vi "ep_Build Waveforms.vi"(0 "AI data":sgl[][](array[numeric]) format="%#.21g", 1 "wiring":T1, 2 "reset? (F)":bool, 5 "AI data channel order":T2[](array[typedef])=[enum."Voltage Phase A (L1)", enum."Voltage Phase B (L2)", enum."Voltage Phase C (L3)", enum."Current Phase A (L1)", enum."Current Phase B (L2)", enum."Current Phase C (L3)", enum."Current Phase N (Neutral)"], 7 "dt":dbl, 9 "t0":timestamp, 11 "error in (no error)":errorcluster) -> (4 "voltage waveforms":waveform(sgl)[](array[waveform]), 6 "current waveforms":waveform(sgl)[](array[waveform]), 15 "error out":errorcluster)   [LabVIEW 2011, in "NI_EP_Power Quality.lvlib"]
uses:
  <vilib>/addons/Electrical Power/PQ/NI_EP_Power Quality.lvlib
  <vilib>/addons/Electrical Power/PQ/Common/Controls/ep_AI Data Channel.ctl
  <vilib>/addons/Electrical Power/PQ/Common/Controls/ep_Wiring.ctl
  <vilib>/addons/Electrical Power/PQ/Scaling_Calibration/subVIs/ep_Compute Third Current (SGL WFM).vi
panel:
  in  "waveform":waveform(sgl)
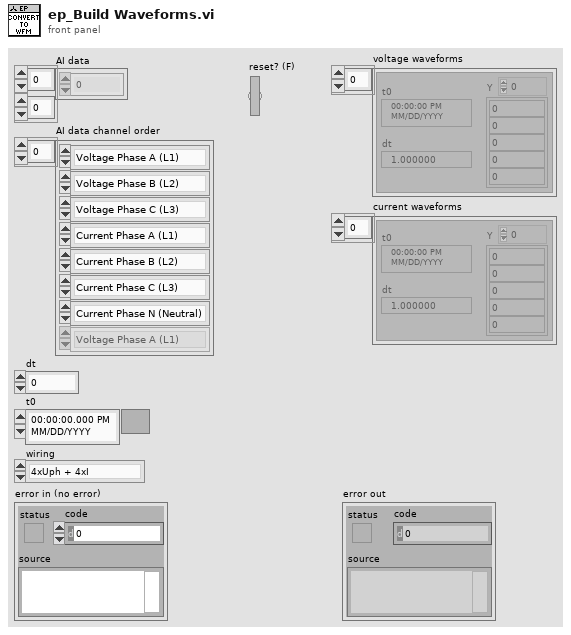
[diagram p1: front panel]
types:
  T1 = typedef "NI_EP_Power Quality.lvlib/ep_Wiring.ctl" = enum16{"4xUph + 4xI", "3xUph + 4xI", "3xUline + 4xI", "3xUph + 3xI", "3xUline + 3xI", "3xUph + 2xI", "3xUline + 2xI", "1xUph + 1xI"}
  T2 = typedef "NI_EP_Power Quality.lvlib/ep_AI Data Channel.ctl" = enum16{"Voltage Phase A (L1)", "Voltage Phase B (L2)", "Voltage Phase C (L3)", "Voltage Phase N (Neutral)", "Current Phase A (L1)", "Current Phase B (L2)", "Current Phase C (L3)", "Current Phase N (Neutral)"}
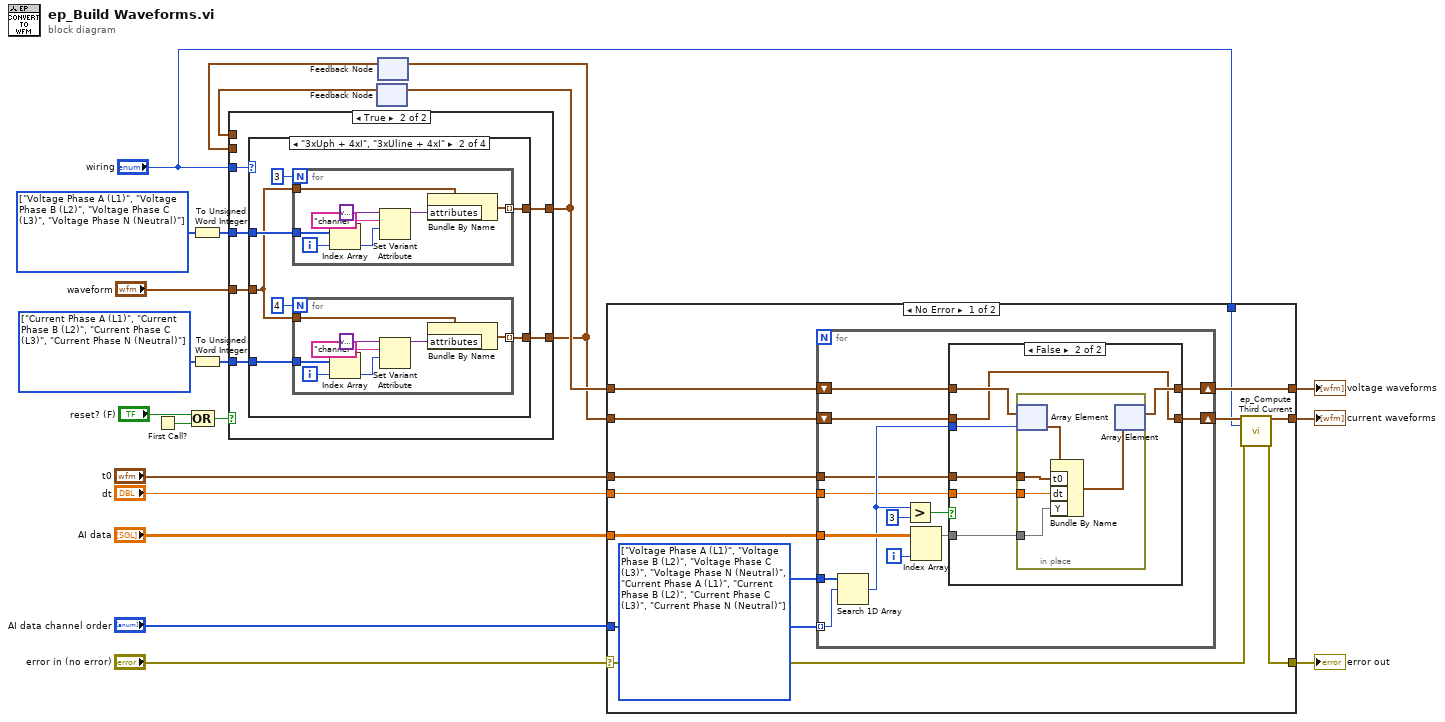
[diagram p0: block diagram]
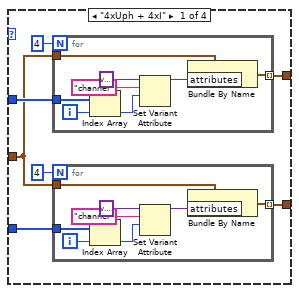
[diagram p3: hidden frame]
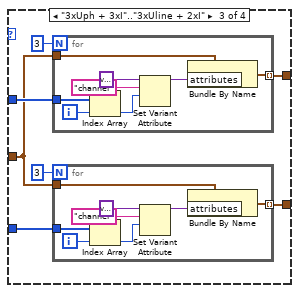
[diagram p4: hidden frame]
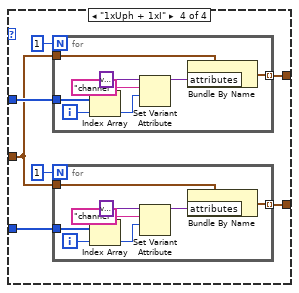
[diagram p5: hidden frame]
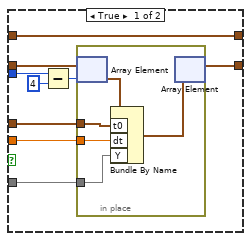
[diagram p6: hidden frame]
diagram:
  w3 = T2[] [enum."Current Phase A (L1)", enum."Current Phase B (L2)", enum."Current Phase C (L3)", enum."Current Phase N (Neutral)"] items=["Voltage Phase A (L1)", "Voltage Phase B (L2)", "Voltage Phase C (L3)", "Voltage Phase N (Neutral)", "Current Phase A (L1)", "Current Phase B (L2)", "Current Phase C (L3)", "Current Phase N (Neutral)"] ("3vol*4cur")
  w5 = T2[] [enum."Voltage Phase A (L1)", enum."Voltage Phase B (L2)", enum."Voltage Phase C (L3)", enum."Voltage Phase N (Neutral)"] items=["Voltage Phase A (L1)", "Voltage Phase B (L2)", "Voltage Phase C (L3)", "Voltage Phase N (Neutral)", "Current Phase A (L1)", "Current Phase B (L2)", "Current Phase C (L3)", "Current Phase N (Neutral)"] ("3vol*4cur")
  n1 = First Call?() -> (First Call?: T/F=w13:bool)
  n2 = To Unsigned Word Integer(number=w5) -> (unsigned 16bit integer=w4:u16[])
  n3 = To Unsigned Word Integer(number=w3) -> (unsigned 16bit integer=w2:u16[])
  n4 = Compound Arithmetic op=OR("reset? (F)", w13) -> (w12:bool)
  n5 = feedback #1() -> (w10:waveform(sgl)[])  [unwired: 1 in]
  n6 = feedback #2() -> (w9:waveform(sgl)[])  [unwired: 1 in]
  n7 = case shown="True" w12 {
    tunnel: "wiring" -> [_ w29]
    tunnel: "waveform" -> [_ w28]
    tunnel: w4 -> [_ w27]
    tunnel: w2 -> [_ w26]
    tunnel: [w22 w25] -> w7
    tunnel: [w23 w24] -> w8
    tunnel: w10 -> [w23 _]
    tunnel: w9 -> [w22 _]
    frame False {
    }
    frame True {
      n8 = case shown="\"3xUph + 4xI\", \"3xUline + 4xI\"" w29 {
        tunnel: w28 -> [w32 w55 w78 w101]
        tunnel: w27 -> [w35 w58 w81 w104]
        tunnel: [w34 w57 w80 w103] -> w24
        tunnel: w26 -> [w31 w54 w77 w100]
        tunnel: [w30 w53 w76 w99] -> w25
        frame "4xUph + 4xI" {
          n9 = for {
            N: 4 -> [_]
            tunnel: w32 -> [w47]
            tunnel: w35 -> [w50]
            tunnel: [w45] -> w34 mode=indexing
            i -> [w49]
            n10 = Index Array(array=w50, index=w49) -> (element=w48:u16)
            n11 = Set Variant Attribute(Variant=variant ("variant"), name="channel", value=w48) -> (Variant out=w46:variant)  [unwired: 1 in, 2 out]
            n12 = Bundle By Name(cluster=w47, "attributes"=w46) -> (w45:waveform(sgl))
          }
          n13 = for {
            N: 4 -> [_]
            tunnel: w32 -> [w40]
            tunnel: [w38] -> w30 mode=indexing
            tunnel: w31 -> [w37]
            i -> [w42]
            n14 = Index Array(array=w37, index=w42) -> (element=w41:u16)
            n15 = Set Variant Attribute(Variant=variant ("variant"), name="channel", value=w41) -> (Variant out=w39:variant)  [unwired: 1 in, 2 out]
            n16 = Bundle By Name(cluster=w40, "attributes"=w39) -> (w38:waveform(sgl))
          }
        }
        frame "3xUph + 4xI", "3xUline + 4xI" {
          n17 = for {
            N: 3 -> [_]
            tunnel: w55 -> [w70]
            tunnel: w58 -> [w73]
            tunnel: [w68] -> w57 mode=indexing
            i -> [w72]
            n18 = Index Array(array=w73, index=w72) -> (element=w71:u16)
            n19 = Set Variant Attribute(Variant=variant ("variant"), name="channel", value=w71) -> (Variant out=w69:variant)  [unwired: 1 in, 2 out]
            n20 = Bundle By Name(cluster=w70, "attributes"=w69) -> (w68:waveform(sgl))
          }
          n21 = for {
            N: 4 -> [_]
            tunnel: w55 -> [w63]
            tunnel: [w61] -> w53 mode=indexing
            tunnel: w54 -> [w60]
            i -> [w65]
            n22 = Index Array(array=w60, index=w65) -> (element=w64:u16)
            n23 = Set Variant Attribute(Variant=variant ("variant"), name="channel", value=w64) -> (Variant out=w62:variant)  [unwired: 1 in, 2 out]
            n24 = Bundle By Name(cluster=w63, "attributes"=w62) -> (w61:waveform(sgl))
          }
        }
        frame "3xUph + 3xI".."3xUline + 2xI" {
          n25 = for {
            N: 3 -> [_]
            tunnel: w78 -> [w93]
            tunnel: w81 -> [w96]
            tunnel: [w91] -> w80 mode=indexing
            i -> [w95]
            n26 = Index Array(array=w96, index=w95) -> (element=w94:u16)
            n27 = Set Variant Attribute(Variant=variant ("variant"), name="channel", value=w94) -> (Variant out=w92:variant)  [unwired: 1 in, 2 out]
            n28 = Bundle By Name(cluster=w93, "attributes"=w92) -> (w91:waveform(sgl))
          }
          n29 = for {
            N: 3 -> [_]
            tunnel: w78 -> [w86]
            tunnel: [w84] -> w76 mode=indexing
            tunnel: w77 -> [w83]
            i -> [w88]
            n30 = Index Array(array=w83, index=w88) -> (element=w87:u16)
            n31 = Set Variant Attribute(Variant=variant ("variant"), name="channel", value=w87) -> (Variant out=w85:variant)  [unwired: 1 in, 2 out]
            n32 = Bundle By Name(cluster=w86, "attributes"=w85) -> (w84:waveform(sgl))
          }
        }
        frame "1xUph + 1xI" {
          n33 = for {
            N: 1 -> [_]
            tunnel: w101 -> [w116]
            tunnel: w104 -> [w119]
            tunnel: [w114] -> w103 mode=indexing
            i -> [w118]
            n34 = Index Array(array=w119, index=w118) -> (element=w117:u16)
            n35 = Set Variant Attribute(Variant=variant ("variant"), name="channel", value=w117) -> (Variant out=w115:variant)  [unwired: 1 in, 2 out]
            n36 = Bundle By Name(cluster=w116, "attributes"=w115) -> (w114:waveform(sgl))
          }
          n37 = for {
            N: 1 -> [_]
            tunnel: w101 -> [w109]
            tunnel: [w107] -> w99 mode=indexing
            tunnel: w100 -> [w106]
            i -> [w111]
            n38 = Index Array(array=w106, index=w111) -> (element=w110:u16)
            n39 = Set Variant Attribute(Variant=variant ("variant"), name="channel", value=w110) -> (Variant out=w108:variant)  [unwired: 1 in, 2 out]
            n40 = Bundle By Name(cluster=w109, "attributes"=w108) -> (w107:waveform(sgl))
          }
        }
      }
    }
  }
  n41 = feedback-in #1(w8) -> ()
  n42 = feedback-in #2(w7) -> ()
  n43 = case shown="No Error" "error in (no error)" {
    selector: "error in (no error)" -> [w123 w175]
    tunnel: [w122 w175] -> w21
    tunnel: "AI data" -> [w134 _]
    tunnel: [w127 _] -> w20
    tunnel: [w125 _] -> w19
    tunnel: "AI data channel order" -> [w133 _]
    tunnel: "t0" -> [w132 _]
    tunnel: "dt" -> [w131 _]
    tunnel: w8 -> [w129 _]
    tunnel: w7 -> [w128 _]
    tunnel: "wiring" -> [w124 _]
    frame No Error {
      w130 = T2[] [enum."Voltage Phase A (L1)", enum."Voltage Phase B (L2)", enum."Voltage Phase C (L3)", enum."Voltage Phase N (Neutral)", enum."Current Phase A (L1)", enum."Current Phase B (L2)", enum."Current Phase C (L3)", enum."Current Phase N (Neutral)"] items=["Voltage Phase A (L1)", "Voltage Phase B (L2)", "Voltage Phase C (L3)", "Voltage Phase N (Neutral)", "Current Phase A (L1)", "Current Phase B (L2)", "Current Phase C (L3)", "Current Phase N (Neutral)"] ("3vol*4cur")
      n44 = for {
        tunnel: w133 -> [w147] mode=indexing
        tunnel: w134 -> [w142]
        shift-right: [w137] -> w127
        shift-left: w129 -> [w146]
        shift-right: [w136] -> w126
        shift-left: w128 -> [w143]
        tunnel: w131 -> [w138]
        tunnel: w132 -> [w139]
        tunnel: w130 -> [w148]
        i -> [w135]
        n45 = Search 1D Array(1D array=w148, element=w147) -> (index of element=w140:i32)  [unwired: 1 in]
        n46 = Greater?(x=w140, y=3) -> (0:w144:bool)
        n47 = Index Array(array=w142, index (col)=w135) -> (element=w141:sgl[])  [unwired: 1 in]
        n48 = case shown="False" w144 {
          tunnel: w146 -> [w151 w166]
          tunnel: w143 -> [w155 w164]
          tunnel: w140 -> [w157 w167]
          tunnel: w141 -> [w149 w163]
          tunnel: w139 -> [w153 w169]
          tunnel: w138 -> [w152 w168]
          tunnel: [w151 w165] -> w137
          tunnel: [w150 w164] -> w136
          frame True {
            n49 = Subtract(x=w157, y=4) -> (x-y=w154:i32)
            n50 = in-place {
              in-place-border: w149 -> [w159]
              in-place-border: w153 -> [w161]
              in-place-border: w152 -> [w160]
              n51 = in-place-array #3(w155, w154) -> (w162:waveform(sgl))
              n52 = Bundle By Name(cluster=w162, "t0"=w161, "dt"=w160, "Y"=w159) -> (w158:waveform(sgl))
              n53 = in-place-array #3(w158) -> (w150:waveform(sgl)[])  [unwired: 1 out]
            }
          }
          frame False {
            n54 = in-place {
              in-place-border: w163 -> [w171]
              in-place-border: w169 -> [w173]
              in-place-border: w168 -> [w172]
              n55 = in-place-array #4(w166, w167) -> (w174:waveform(sgl))
              n56 = Bundle By Name(cluster=w174, "t0"=w173, "dt"=w172, "Y"=w171) -> (w170:waveform(sgl))
              n57 = in-place-array #4(w170) -> (w165:waveform(sgl)[])  [unwired: 1 out]
            }
          }
        }
      }
      n58 = call-poly <vilib>:"ep_Compute Third Current.vi"("current waveforms in"=w126, "wiring"=w124, "error in (no error)"=w123) -> ("current waveforms out"=w125:waveform(sgl)[], "error out"=w122:errorcluster)  [unwired: 11 in]
    }
    frame Error {
    }
  }
  "voltage waveforms" <- w20
  "error out" <- w21
  "current waveforms" <- w19
